vi "3-4.vi"(2 "字符串 2":string, 3 "输入 1":dbl, 4 "字符串":string) -> (0 "长度":i32, 1 "连接的字符串":string)   [LabVIEW 2017]
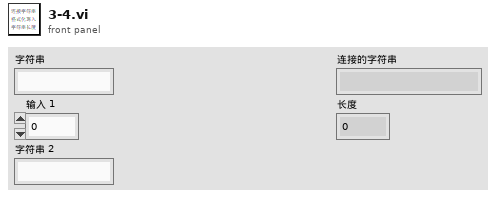
[diagram p1: front panel]
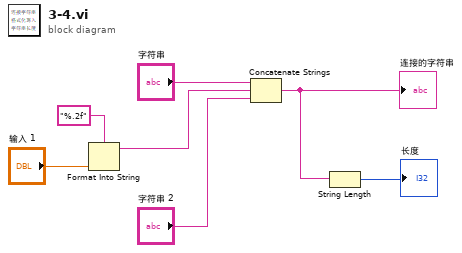
[diagram p0: block diagram]
diagram:
  n1 = Format Into String(format string="%.2f" ("格式字符串"), "输入 1") -> (resulting string=w5:string)  [unwired: 2 in, 1 out]
  n2 = Concatenate Strings("字符串", w5, "字符串 2") -> (w3:string)
  "连接的字符串" <- w3
  n3 = String Length(string=w3) -> (length=→"长度":i32)
